vi "Tag Based Metadata Start.vi"(0 "Metadata Save Path":path, 7 "Preload Metadata":path, 11 "Error In":errorcluster) -> (15 "Error Out":errorcluster)   [LabVIEW 2020]
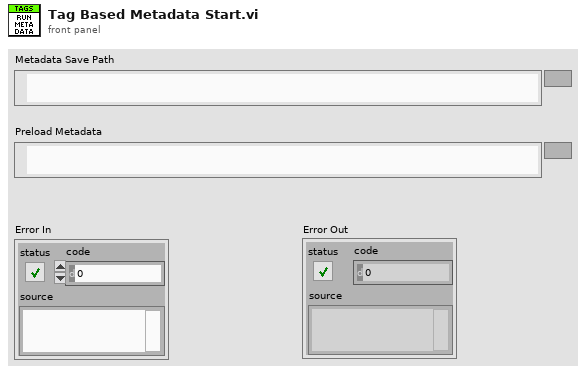
[diagram p1: front panel]
types:
  T1 = enum32{"Invalid", "Standard", "Closed", "Hidden", "Minimized", "Maximized"}
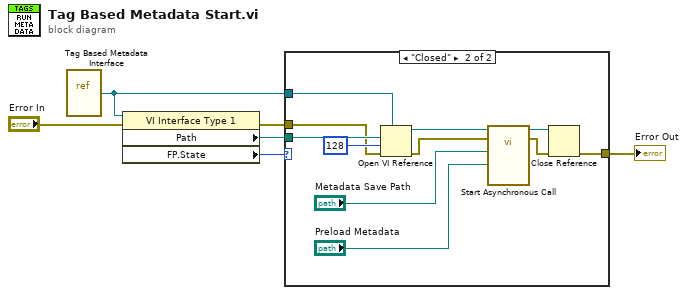
[diagram p0: block diagram]
diagram:
  n1 = vi-ref "Tag Based Metadata Interface.vi"() -> (w6:refnum<vi>)
  n2 = property class="VI Interface Type 1"(reference=w6, error in="Error In") -> (error out=w3:errorcluster, "Path"=w5:path, "FP.State"=w4:T1)  [unwired: 1 out]
  n3 = case shown="\"Closed\"" w4 {
    tunnel: w6 -> [_ w16]
    tunnel: w5 -> [_ w15]
    tunnel: w3 -> [w7 w13]
    tunnel: [w7 w10] -> w2
    frame Default {
    }
    frame "Closed" {
      n4 = Open VI Reference(type specifier VI Refnum (for type only)=w16, vi path=w15, options=128, error in (no error)=w13) -> (vi reference=w17:refnum<vi>, error out=w12:errorcluster)  [unwired: 2 in]
      n5 = call-by-ref "Start Asynchronous Call"(reference=w17, error in=w12, "Save Path"="Metadata Save Path", "Input Tags"="Preload Metadata") -> (reference out=w18:refnum<vi>, error out=w11:errorcluster)  [unwired: 14 in]
      n6 = Close Reference(reference=w18, error in (no error)=w11) -> (error out=w10:errorcluster)
    }
  }
  "Error Out" <- w2
